vi "CRAB and II.vi"() -> ()   [LabVIEW 2017]
uses:
  <vilib>/Instr/_visa.llb/VISA Configure Serial Port (Instr).vi
  <instrlib>/BK Precision 913XX/BK Precision 913XX.lvlib
panel:
  in  "Send 4":bool
  out "Message":string
  in  "Reset 4":bool
  out "HV On":bool
  out "Fault":bool
  out "Vmode 4":bool
  out "Imode 4":bool
  out "Voltage Monitor":dbl format="%#.2g"
  out "Current Monitor":dbl format="%#.2g"
  in  "High Voltage":bool
  in  "Voltage Program":dbl min=0.0 max=100.0 step=0.1 format="%#.2g"
  in  "Current Program":dbl min=0.0 max=100.0 step=0.1 format="%#.2g"
  in  "Version 4":bool
  in  "?":bool
  in  "Baud Rate":u16=9600 min=1200 max=19200 step=1200
  in  "Flow Control":u16(ring) items=["None"=0, "XON/XOFF"=1, "RTS/CTS"=2, "DTR/DSR"=4]
  in  "Stop Bits":u16(ring)=10 items=["1.0"=10, "1.5"=15, "2.0"=20]
  in  "Parity":u16(ring) items=["None", "Odd", "Even", "Mark", "Space"]
  in  "Data Bits":u16=8 min=5 max=8 step=1
  in  "VISA resource name":refnum<visa-resource-name>="COM1"
  out "Current Monitor 1":dbl format="%.4g"
  out "Power Monitor 1":dbl format="%.4g"
  out "Voltage Monitor 1":dbl format="%.4g"
  out "Current Monitor 2":dbl format="%.4g"
  out "Power Monitor 2":dbl format="%.4g"
  out "Voltage Monitor 2":dbl format="%.4g"
  out "Current Monitor 3":dbl format="%.4g"
  out "Power Monitor 3":dbl format="%.4g"
  out "Voltage Monitor 3":dbl format="%.4g"
  in  "Voltage Level (0.0 V)":dbl format="%.3g"
  in  "Voltage Level (0.0 V) 2":dbl format="%.3g"
  in  "Voltage Level (0.0 V) 3":dbl format="%.3g"
  in  "Channel (3:3)":u16(ring)=1 items=["1"=1, "2"=2, "3"=3]
  in  "Channel (2:2)":u16(ring)=1 items=["1"=1, "2"=2, "3"=3]
  in  "Channel (1:1)":u16(ring)=1 items=["1"=1, "2"=2, "3"=3]
  in  "Enable OVP":bool=TRUE
  in  "Stop Output":bool
  in  "Voltage Limit":dbl=36.0 min=0.0 max=66.0 step=0.001 format="%.3g"
  in  "Current Limit":dbl min=0.0 max=25.0 step=1.0 format="%.3f"
  in  "VISA resource name":refnum<visa-resource-name>
  in  "Send 3":bool
  out "Message":string
  in  "Reset 3":bool
  out "HV On":bool
  out "Fault":bool
  out "Vmode 3":bool
  out "Imode 3":bool
  out "Voltage Monitor":dbl format="%#.2g"
  out "Current Monitor":dbl format="%#.2g"
  in  "High Voltage":bool
  in  "Voltage Program":dbl min=0.0 max=100.0 step=0.1 format="%#.2g"
  in  "Current Program":dbl min=0.0 max=100.0 step=0.1 format="%#.2g"
  in  "Version 3":bool
  in  "?":bool
  in  "Baud Rate":u16=9600 min=1200 max=19200 step=1200
  in  "Flow Control":u16(ring) items=["None"=0, "XON/XOFF"=1, "RTS/CTS"=2, "DTR/DSR"=4]
  in  "Stop Bits":u16(ring)=10 items=["1.0"=10, "1.5"=15, "2.0"=20]
  in  "Parity":u16(ring) items=["None", "Odd", "Even", "Mark", "Space"]
  in  "Data Bits":u16=8 min=5 max=8 step=1
  in  "VISA resource name":refnum<visa-resource-name>="COM1"
  in  "Send":bool
  in  "Reset":bool
  in  "High Voltage":bool
  in  "Voltage Program":dbl min=0.0 max=100.0 step=0.1 format="%#.2g"
  in  "Current Program":dbl min=0.0 max=100.0 step=0.1 format="%#.2g"
  in  "Version":bool
  in  "?":bool
  in  "Baud Rate":u16=9600 min=1200 max=19200 step=1200
  in  "Flow Control":u16(ring) items=["None"=0, "XON/XOFF"=1, "RTS/CTS"=2, "DTR/DSR"=4]
  in  "Stop Bits":u16(ring)=10 items=["1.0"=10, "1.5"=15, "2.0"=20]
  in  "Parity":u16(ring) items=["None", "Odd", "Even", "Mark", "Space"]
  in  "Data Bits":u16=8 min=5 max=8 step=1
  in  "VISA resource name":refnum<visa-resource-name>="COM1"
  out "Message":string
  out "HV On":bool
  out "Fault":bool
  out "Vmode":bool
  out "Imode":bool
  out "Voltage Monitor":dbl format="%#.2g"
  out "Current Monitor":dbl format="%#.2g"
  # "LabVIEW Instructions: READ ALL INSTRUCTIONS BEFORE OPERATING\n\n1) Set all VISA resource names to their appropiate settings (Labeled & color coded)\n2)Flip HV switch from off to on.\n3) Start program (white arrow on top left). Green \"Voltage Monitor\" light should turn on in the corresponding monitors.  \n4) Read individual insturctions for each region (II, FC, EL) and send voltage programs.Once you send the voltage programs, the red \"HV on\" lights should turn on.\n\n  Now, you are ready to operate CRAB! \n\nNote: You shouldn't have to touch any of the configuration settings, only edit programs!"
  # "I I CONTROLS"
  # "EL + CONTROLS"
  # "FIELD CAGE CONTROLS"
  # "Configuration"
  # "Configuration"
  # "Configuration"
  # "EL+ Instructions:\n\nSet VISA resource name to COM6.\n\nTo start: Set Voltage to 2kV & Current to 0.1 amps\n\nVoltage goes up to 8kV. Slow ramp from 4-8kV in increments of .5kV every ~30 seconds. DO NOT EXCEED 8 KV WHEN OPERATING CRAB"
  # "Programs"
  # "Programs"
  # "Programs"
  # "On"
  # "On"
  # "kV"
  # "kV"
  # "[ppsjgsln"
  # "Image Intesnifier Instructions:\n\nSet VISA resource name to USB::0XFFF::0X913....::instr\n\nSet channels accordingly (ie Channel 2 to 2). \n\nSet Voltage limit to 6 and Current limit to 1.   ENSURE OVER VOLTAGE PROTECION (OVP) IS ENABLED. This will apply on the Voltage limit, so you do not need to worry about exceeding voltage (you will get an error and a beep if you do)"
  # "V"
  # "V"
  # "V"
  # "A"
  # "Off"
  # "Off"
  # "A"
  # "EL ++ CONTROLS"
  # "EL++ Instructions:\n\nSet VISA resource name to COM4.\n\nTo start: Set Voltage to 2kV & Current to 0.1 amps\n\nVoltage goes up to 15kV. Slow ramp from 4-15kV in increments of .5kV every ~30 seconds. DO NOT EXCEED 18 KV WHEN OPERATING CRAB"
  # "Field Cage Instructions:\n\nSet VISA resource name to COM8.\n\nTo start: Set Voltage to 2kV & Current to 0.1 amps\n\nVoltage goes up to 7kV.\nSlow ramp from 4-7kV in increments of .5kV every ~30 seconds. DO NOT EXCEED 8 KV WHEN OPERATING CRAB"
  # "Monitors"
  # "Monitors"
  # "Monitors"
  # "Configuration"
  # "V"
  # "V"
  # "V"
  # "kV"
  # "kV"
  # "V"
  # "V"
  # "V"
  # "A"
  # "A"
  # "Programs"
  # "V"
  # "V"
  # "V"
  # "On"
  # "kV"
  # "Off"
  # "A"
  # "IMAGE INTENSIFIER REGION"
  # "Monitors"
  # "kV"
  # "FIELD CAGE REGION"
  # "A"
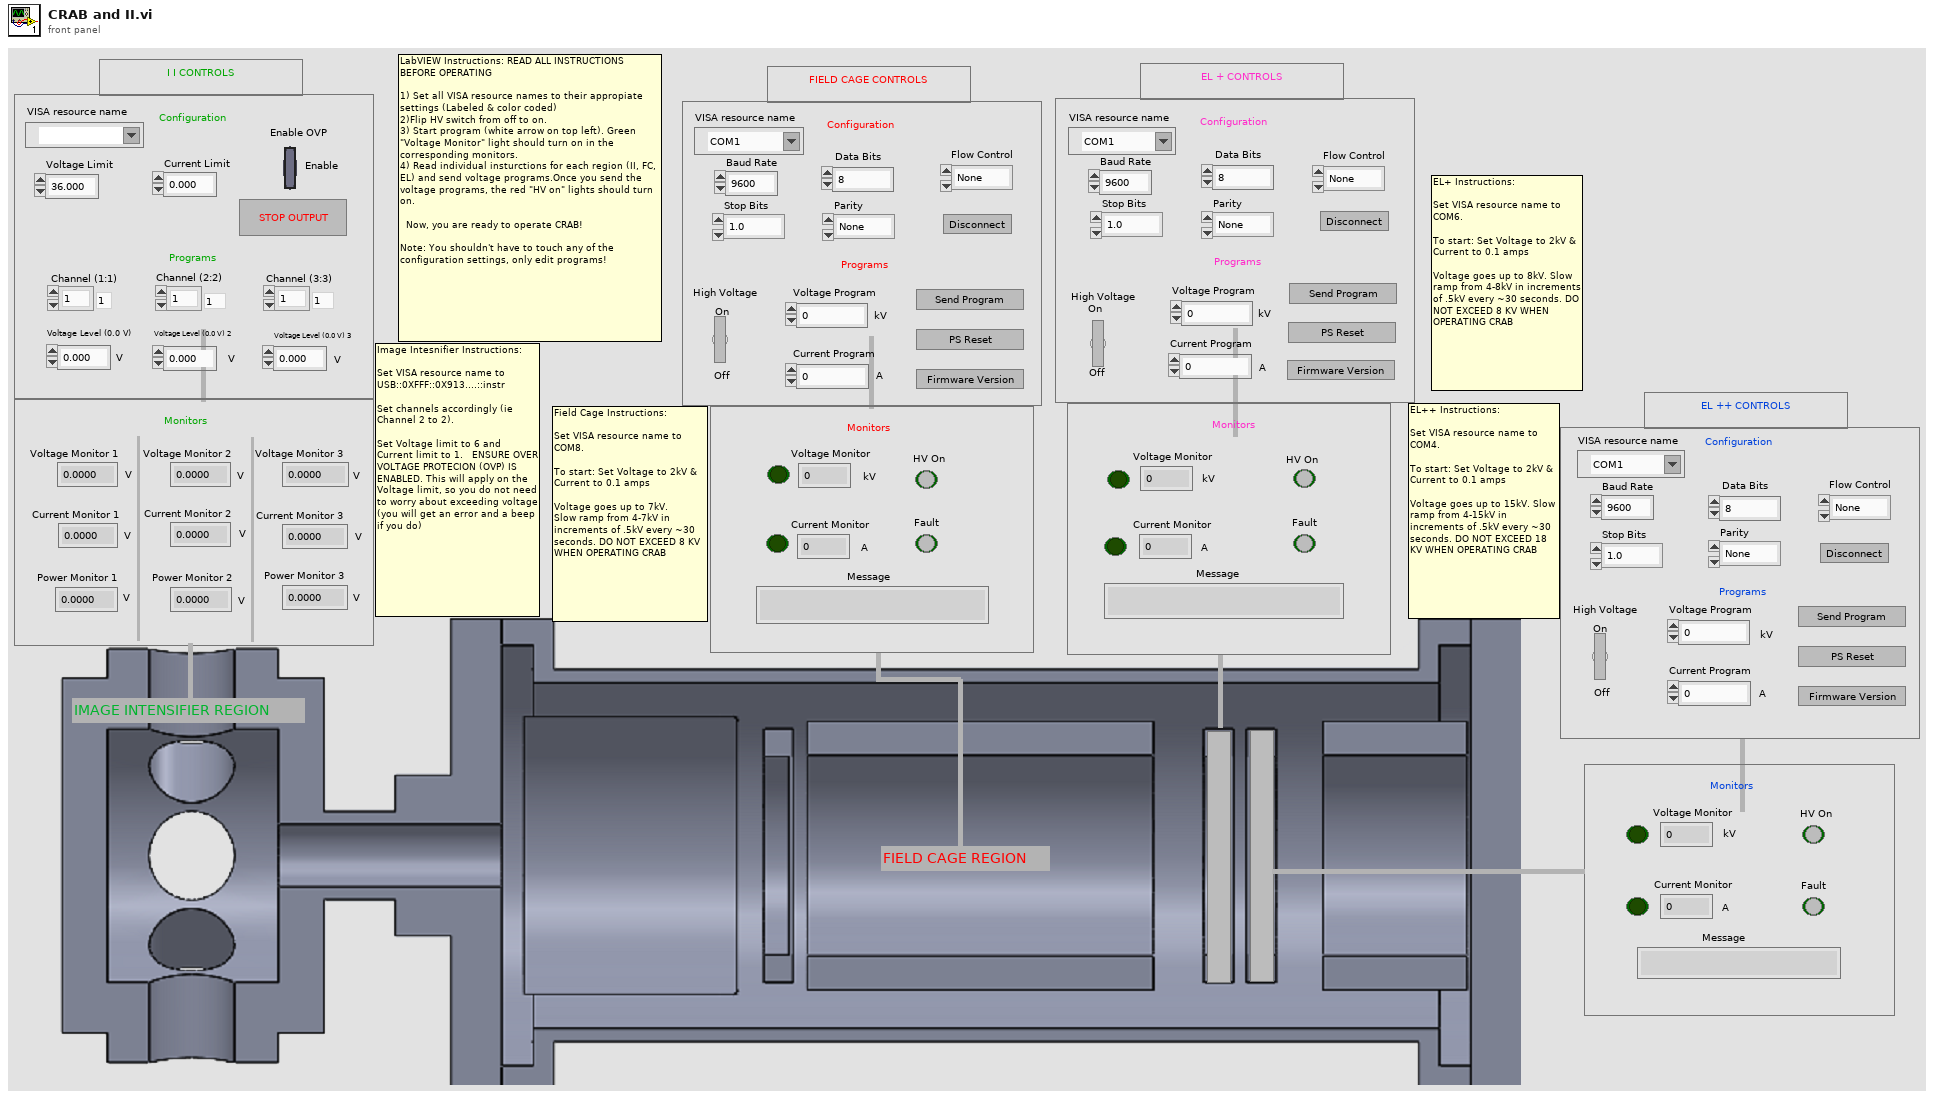
[diagram p1: front panel]
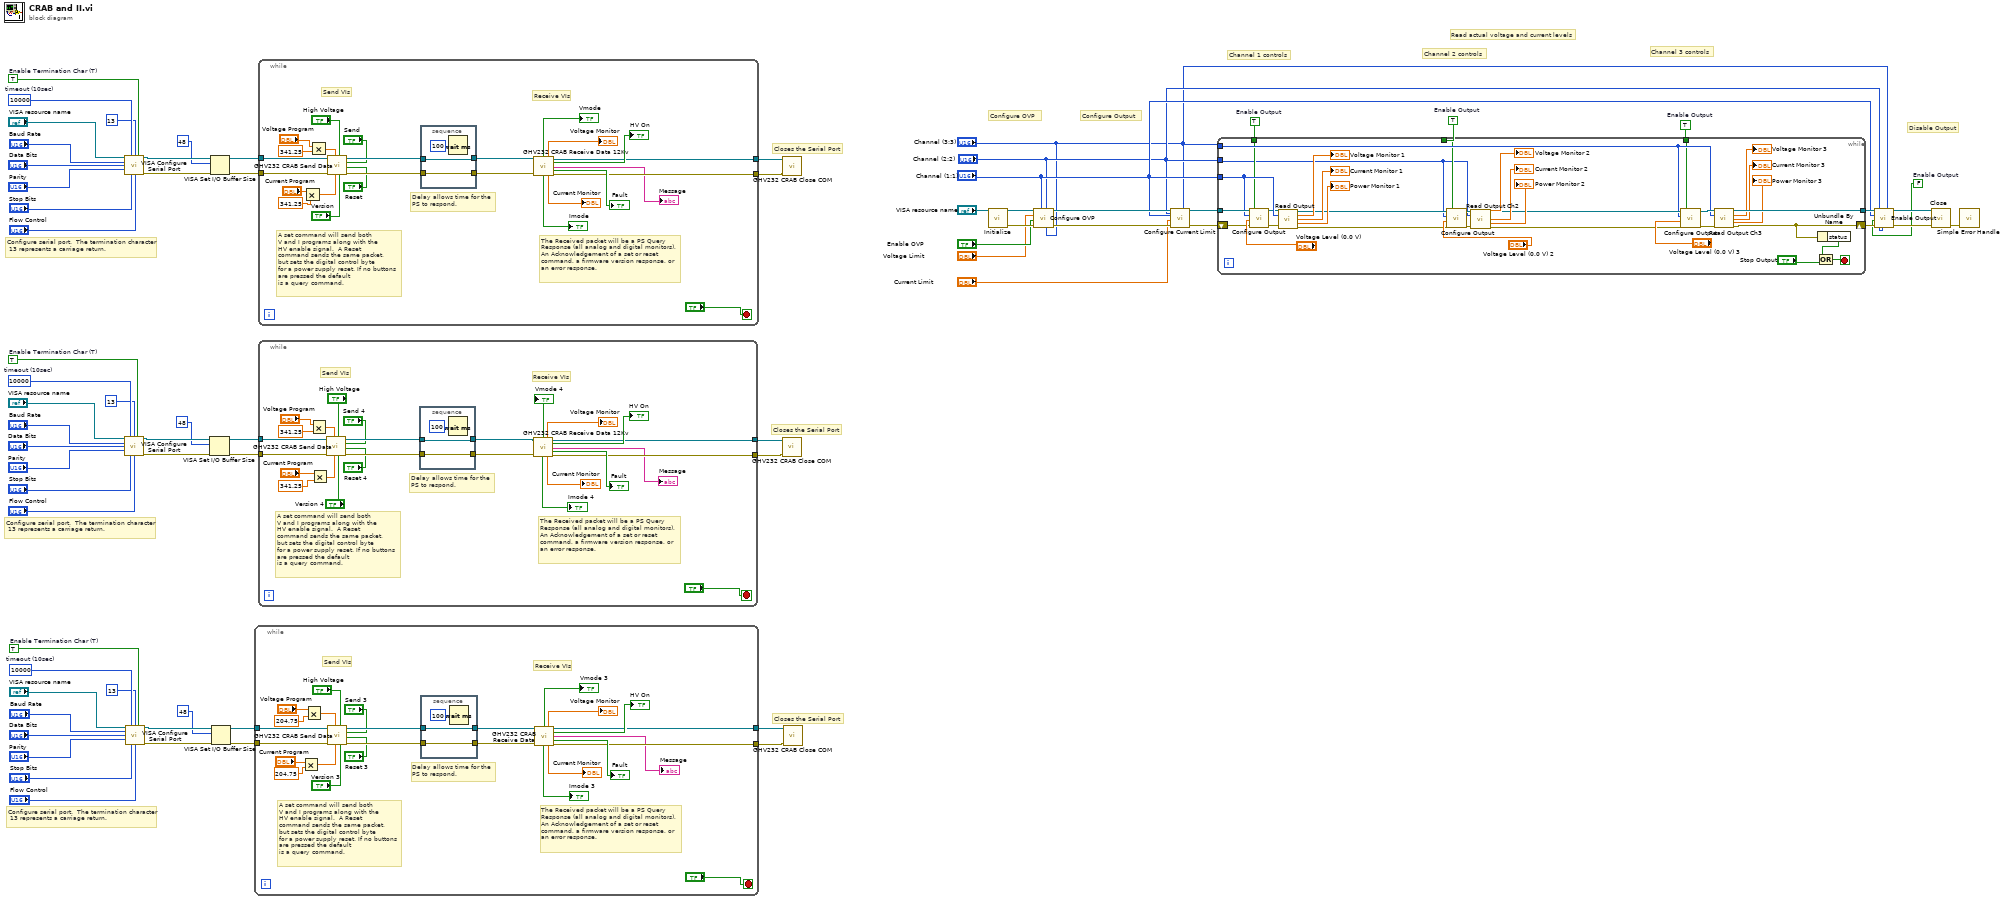
[diagram p0: block diagram]
diagram:
  w13 = TRUE  # Enable Termination Char (T)
  w14 = u32 10000  # timeout (10sec)
  w19 = TRUE  # Enable Output
  w20 = TRUE  # Enable Output
  w21 = TRUE  # Enable Output
  w23 = FALSE  # Enable Output
  w51 = TRUE  # Enable Termination Char (T)
  w52 = u32 10000  # timeout (10sec)
  w67 = TRUE  # Enable Termination Char (T)
  w68 = u32 10000  # timeout (10sec)
  # "Closes the Serial Port"
  # "Configure serial port.  The termination character\n 13 represents a carriage return."
  # "Channel 3 controls"
  # "Channel 2 controls"
  # "Channel 1 controls"
  # "Disable Output"
  # "Read actual voltage and current levels"
  # "Configure Output"
  # "Configure OVP"
  # "Closes the Serial Port"
  # "Configure serial port.  The termination character\n 13 represents a carriage return."
  # "Closes the Serial Port"
  # "Configure serial port.  The termination character\n 13 represents a carriage return."
  n1 = call-poly "VISA Configure Serial Port"("VISA resource name"="VISA resource name", "timeout (10sec)"=w14, "termination char\n(0xA = '\\n' = LF)"=13, "Enable Termination\nChar (T)"=w13, "baud rate (9600)"="Baud Rate", "data bits (8)"="Data Bits", "parity (0:none)"="Parity", "stop bits (10: 1 bit)"="Stop Bits", "flow control (0:none)"="Flow Control") -> ("VISA resource name out"=w3:refnum<visa-resource-name>, "error out"=w2:errorcluster)  [unwired: 5 in]
  n2 = call-poly "VISA Configure Serial Port"("VISA resource name"="VISA resource name", "timeout (10sec)"=w68, "termination char\n(0xA = '\\n' = LF)"=13, "Enable Termination\nChar (T)"=w67, "baud rate (9600)"="Baud Rate", "data bits (8)"="Data Bits", "parity (0:none)"="Parity", "stop bits (10: 1 bit)"="Stop Bits", "flow control (0:none)"="Flow Control") -> ("VISA resource name out"=w57:refnum<visa-resource-name>, "error out"=w56:errorcluster)  [unwired: 5 in]
  n3 = call-poly "VISA Configure Serial Port"("VISA resource name"="VISA resource name", "timeout (10sec)"=w52, "termination char\n(0xA = '\\n' = LF)"=13, "Enable Termination\nChar (T)"=w51, "baud rate (9600)"="Baud Rate", "data bits (8)"="Data Bits", "parity (0:none)"="Parity", "stop bits (10: 1 bit)"="Stop Bits", "flow control (0:none)"="Flow Control") -> ("VISA resource name out"=w41:refnum<visa-resource-name>, "error out"=w40:errorcluster)  [unwired: 5 in]
  n4 = VISA Set I/O Buffer Size(VISA resource name=w3, mask (16)=48, error in (no error)=w2) -> (VISA resource name out=w4:refnum<visa-resource-name>, error out=w5:errorcluster)  [unwired: 1 in]
  n5 = VISA Set I/O Buffer Size(VISA resource name=w57, mask (16)=48, error in (no error)=w56) -> (VISA resource name out=w58:refnum<visa-resource-name>, error out=w59:errorcluster)  [unwired: 1 in]
  n6 = VISA Set I/O Buffer Size(VISA resource name=w41, mask (16)=48, error in (no error)=w40) -> (VISA resource name out=w42:refnum<visa-resource-name>, error out=w43:errorcluster)  [unwired: 1 in]
  n7 = while {
    tunnel: w43 -> [w94]
    tunnel: w42 -> [w93]
    tunnel: [w83] -> w45
    tunnel: [w79] -> w44
    stop <- "?" stop-if-true
    # "The Received packet will be a PS Query\nResponse (all analog and digital monitors),\nAn Acknowledgement of a set or reset\ncommand, a firmware version response, or\nan error response."
    # "Delay allows time for the \nPS to respond."
    # "A set command will send both\nV and I programs along with the\nHV enable signal.  A Reset \ncommand sends the same packet,\nbut sets the digital control byte\nfor a power supply reset. If no buttons are pressed the default\nis a query command."
    # "Receive VIs"
    # "Send VIs"
    n8 = Multiply(x="Current Program", y=204.75) -> (x*y=w71:dbl)
    n9 = Multiply(x="Voltage Program", y=204.75) -> (x*y=w74:dbl)
    n10 = call "GHV232 CRAB Send Data.vi"("Reset"="Reset 3", "Send"="Send 3", "Version"="Version 3", "HV Enable"="High Voltage", "Current Program"=w71, "Voltage Program"=w74, "error in (no error)"=w94, "VISA resource name"=w93) -> ("error out"=w96:errorcluster, "VISA resource name 2"=w95:refnum<visa-resource-name>)  [unwired: 2 in]
    n11 = stacked-sequence {
      tunnel: [w99] -> w88
      tunnel: w95 -> [w99]
      tunnel: w96 -> [w98]
      tunnel: [w98] -> w87
      frame #0 {
        n12 = Wait (ms)(milliseconds to wait=100) -> ()  [unwired: 1 out]
      }
    }
    n13 = call "GHV232 CRAB Receive Data.vi"("VISA resource name"=w88, "error in (no error)"=w87) -> ("V"=→"Vmode 3":bool, "Vmon"=→"Voltage Monitor":dbl, "VISA resource name 2"=w83:refnum<visa-resource-name>, "HV on"=→"HV On":bool, "Message"=→"Message":string, "Fault"=→"Fault":bool, "I"=→"Imode 3":bool, "Imon"=→"Current Monitor":dbl, "error out"=w79:errorcluster)  [unwired: 5 in]
  }
  n14 = while {
    tunnel: w5 -> [w123]
    tunnel: w4 -> [w122]
    tunnel: [w113] -> w7
    tunnel: [w109] -> w6
    stop <- "?" stop-if-true
    # "The Received packet will be a PS Query\nResponse (all analog and digital monitors),\nAn Acknowledgement of a set or reset\ncommand, a firmware version response, or\nan error response."
    # "Delay allows time for the \nPS to respond."
    # "A set command will send both\nV and I programs along with the\nHV enable signal.  A Reset \ncommand sends the same packet,\nbut sets the digital control byte\nfor a power supply reset. If no buttons are pressed the default\nis a query command."
    # "Receive VIs"
    # "Send VIs"
    n15 = Multiply(x="Voltage Program", y=341.25) -> (x*y=w106:dbl)
    n16 = Multiply(x="Current Program", y=341.25) -> (x*y=w103:dbl)
    n17 = call "GHV232 CRAB Send Data.vi"("Reset"="Reset 4", "Send"="Send 4", "Version"="Version 4", "HV Enable"="High Voltage", "Current Program"=w103, "Voltage Program"=w106, "error in (no error)"=w123, "VISA resource name"=w122) -> ("error out"=w125:errorcluster, "VISA resource name 2"=w124:refnum<visa-resource-name>)  [unwired: 2 in]
    n18 = stacked-sequence {
      tunnel: [w128] -> w117
      tunnel: w124 -> [w128]
      tunnel: w125 -> [w127]
      tunnel: [w127] -> w116
      frame #0 {
        n19 = Wait (ms)(milliseconds to wait=100) -> ()  [unwired: 1 out]
      }
    }
    n20 = call "GHV232 CRAB Receive Data 12Kv.vi"("VISA resource name"=w117, "error in (no error)"=w116) -> ("V"=→"Vmode 4":bool, "Vmon"=→"Voltage Monitor":dbl, "VISA resource name 2"=w113:refnum<visa-resource-name>, "HV on"=→"HV On":bool, "Message"=→"Message":string, "Fault"=→"Fault":bool, "I"=→"Imode 4":bool, "Imon"=→"Current Monitor":dbl, "error out"=w109:errorcluster)  [unwired: 5 in]
  }
  n21 = while {
    tunnel: w59 -> [w152]
    tunnel: w58 -> [w151]
    tunnel: [w141] -> w61
    tunnel: [w137] -> w60
    stop <- "?" stop-if-true
    # "The Received packet will be a PS Query\nResponse (all analog and digital monitors),\nAn Acknowledgement of a set or reset\ncommand, a firmware version response, or\nan error response."
    # "Delay allows time for the \nPS to respond."
    # "A set command will send both\nV and I programs along with the\nHV enable signal.  A Reset \ncommand sends the same packet,\nbut sets the digital control byte\nfor a power supply reset. If no buttons are pressed the default\nis a query command."
    # "Receive VIs"
    # "Send VIs"
    n22 = Multiply(x="Current Program", y=341.25) -> (x*y=w129:dbl)
    n23 = Multiply(x="Voltage Program", y=341.25) -> (x*y=w132:dbl)
    n24 = call "GHV232 CRAB Send Data.vi"("Reset"="Reset", "Send"="Send", "Version"="Version", "HV Enable"="High Voltage", "Current Program"=w129, "Voltage Program"=w132, "error in (no error)"=w152, "VISA resource name"=w151) -> ("error out"=w154:errorcluster, "VISA resource name 2"=w153:refnum<visa-resource-name>)  [unwired: 2 in]
    n25 = stacked-sequence {
      tunnel: [w157] -> w146
      tunnel: w153 -> [w157]
      tunnel: w154 -> [w156]
      tunnel: [w156] -> w145
      frame #0 {
        n26 = Wait (ms)(milliseconds to wait=100) -> ()  [unwired: 1 out]
      }
    }
    n27 = call "GHV232 CRAB Receive Data 12Kv.vi"("VISA resource name"=w146, "error in (no error)"=w145) -> ("V"=→"Vmode":bool, "Vmon"=→"Voltage Monitor":dbl, "VISA resource name 2"=w141:refnum<visa-resource-name>, "HV on"=→"HV On":bool, "Message"=→"Message":string, "Fault"=→"Fault":bool, "I"=→"Imode":bool, "Imon"=→"Current Monitor":dbl, "error out"=w137:errorcluster)  [unwired: 5 in]
  }
  n28 = call "GHV232 CRAB Close COM.vi"("error in (no error)"=w6, "VISA resource name"=w7) -> ()  [unwired: 9 in, 1 out]
  n29 = call "GHV232 CRAB Close COM.vi"("error in (no error)"=w60, "VISA resource name"=w61) -> ()  [unwired: 9 in, 1 out]
  n30 = call "GHV232 CRAB Close COM.vi"("error in (no error)"=w44, "VISA resource name"=w45) -> ()  [unwired: 9 in, 1 out]
  n31 = call <instrlib>:"Initialize.vi"("VISA resource name"="VISA resource name") -> ("error out"=w36:errorcluster, "VISA resource name out"=w35:refnum<visa-resource-name>)  [unwired: 9 in]
  n32 = call <instrlib>:"Configure OVP.vi"("Channel (3:3)"="Channel (3:3)", "Channel (2:2)"="Channel (2:2)", "Channel (1:1)"="Channel (1:1)", "error in (no error)"=w36, "Enable OVP (T: Enable)"="Enable OVP", "Voltage Limit (36.000 V)"="Voltage Limit", "VISA resource name"=w35) -> ("error out"=w33:errorcluster, "VISA resource name out"=w34:refnum<visa-resource-name>)  [unwired: 3 in]
  n33 = call <instrlib>:"Configure Current Limit.vi"("Channel (3:3)"="Channel (3:3)", "Channel (2:2)"="Channel (2:2)", "error in (no error)"=w33, "Current Limit (0.0 A)"="Current Limit", "Channel (1:1)"="Channel (1:1)", "VISA resource name"=w34) -> ("error out"=w29:errorcluster, "VISA resource name out"=w28:refnum<visa-resource-name>)  [unwired: 4 in]
  n34 = while {
    tunnel: w28 -> [w186]
    tunnel: [w183] -> w32
    shift-right: [w159] -> w27
    shift-left: w29 -> [w165]
    tunnel: "Channel (1:1)" -> [w185]
    tunnel: "Channel (2:2)" -> [w158]
    tunnel: "Channel (3:3)" -> [w172]
    tunnel: w21 -> [w171]
    tunnel: w20 -> [w167]
    tunnel: w19 -> [w170]
    stop <- w192 stop-if-true
    n35 = call <instrlib>:"Configure Output.vi"("Enable Channel Output (F: False)"=w171, "error in (no error)"=w165, "Voltage Level (0.0 V)"="Voltage Level (0.0 V)", "Channel (1:1)"=w185, "VISA resource name"=w186) -> ("error out"=w164:errorcluster, "VISA resource name out"=w175:refnum<visa-resource-name>)  [unwired: 5 in]
    n36 = call <instrlib>:"Read Output.vi"("VISA resource name"=w175, "Channel (1:Channel 1)"=w185, "error in (no error)"=w164) -> ("VISA resource name out"=w168:refnum<visa-resource-name>, "Actual Voltage Level (V)"=→"Voltage Monitor 1":dbl, "Actual Current Level (A)"=→"Current Monitor 1":dbl, "Actual Power Level (W)"=→"Power Monitor 1":dbl, "error out"=w163:errorcluster)  [unwired: 8 in]
    n37 = call <instrlib>:"Configure Output.vi"("Enable Channel Output (F: False)"=w167, "error in (no error)"=w163, "Voltage Level (0.0 V)"="Voltage Level (0.0 V) 2", "Channel (1:1)"=w158, "VISA resource name"=w168) -> ("error out"=w162:errorcluster, "VISA resource name out"=w169:refnum<visa-resource-name>)  [unwired: 5 in]
    n38 = call <instrlib>:"Read Output Ch2.vi"("VISA resource name"=w169, "Channel (1:Channel 1)"=w158, "error in (no error)"=w162) -> ("VISA resource name out"=w174:refnum<visa-resource-name>, "Actual Voltage Level (V)"=→"Voltage Monitor 2":dbl, "Actual Current Level (A)"=→"Current Monitor 2":dbl, "Actual Power Level (W)"=→"Power Monitor 2":dbl, "error out"=w161:errorcluster)  [unwired: 8 in]
    n39 = call <instrlib>:"Configure Output.vi"("Enable Channel Output (F: False)"=w170, "error in (no error)"=w161, "Voltage Level (0.0 V)"="Voltage Level (0.0 V) 3", "Channel (1:1)"=w172, "VISA resource name"=w174) -> ("error out"=w160:errorcluster, "VISA resource name out"=w173:refnum<visa-resource-name>)  [unwired: 5 in]
    n40 = call <instrlib>:"Read Output Ch3.vi"("VISA resource name"=w173, "Channel (1:Channel 1)"=w172, "error in (no error)"=w160) -> ("VISA resource name out"=w183:refnum<visa-resource-name>, "Actual Voltage Level (V)"=→"Voltage Monitor 3":dbl, "Actual Current Level (A)"=→"Current Monitor 3":dbl, "Actual Power Level (W)"=→"Power Monitor 3":dbl, "error out"=w159:errorcluster)  [unwired: 8 in]
    n41 = Unbundle By Name(w159) -> ("status"=w190:bool)
    n42 = Or(x=w190, y="Stop Output") -> (x .or. y?=w192:bool)
  }
  n43 = call <instrlib>:"Enable Output.vi"("Channel (3:3)"="Channel (3:3)", "Channel (2:2)"="Channel (2:2)", "error in (no error)"=w27, "Enable Output (F: False)"=w23, "Channel (1:1)"="Channel (1:1)", "VISA resource name"=w32) -> ("error out"=w30:errorcluster, "VISA resource name out"=w31:refnum<visa-resource-name>)  [unwired: 4 in]
  n44 = call <instrlib>:"Close.vi"("error in (no error)"=w30, "VISA resource name"=w31) -> ("error out"=w37:errorcluster)  [unwired: 9 in]
  n45 = call <vilib>:"Simple Error Handler.vi"("error in (no error)"=w37) -> ()  [unwired: 4 in, 5 out]
